vi "AO_6711_Init_Session.vi"(8 "error in (no error)":errorcluster, 9 "TRAPPING Inputs":T1={"Number of Channels"=4, "Init Values"=[2.0, 9.0, 2.0, 9.0], "Opening Values"=[0.0, 0.0, 0.0, 0.0], "Trapping Values"=[2.0, 9.0, 2.0, 9.0], "Emptying Values"=[-10.0, -10.0, -10.0, -10.0], "Adiabatic ON"=FALSE, "Adiabatic Duration"=100, "Adiabatic Waveforms"=["Adiabatic_None_2_2_2000", "Adiabatic_Ramp_9_0_2000", "Adiabatic_None_2_2_2000", "Adiabatic_RC_9_0_2000"], "Ions Refill ON"=FALSE, "Number of Ions Refills"=1} {"Number of Ions Refills" min=1 max=1000; "Trapping Values" min=-10.0 max=10.0; "Init Values" min=-10.0 max=10.0; "Emptying Values" min=-10.0 max=10.0; "Opening Values" min=-10.0 max=10.0}, 10 "AO 6711 Inputs":T2={"Physical Channels"="AO_6711/ao0:3", "Min Voltage"=-10.0, "Max Voltage"=10.0, "Trigger Source"="/AO_6711/PFI3", "Counter"="AO_6711/ctr0"} {"Max Voltage" min=-10.0 max=10.0; "Min Voltage" min=-10.0 max=10.0}, 11 "Use Software Trigger":bool) -> (0 "error out":errorcluster, 3 "Instrument handle out":refnum<k21>)   [LabVIEW 2020]
doc: "This VI inits a waveform generation session for the AO6711 board.\n1. The physical channels are selected as Analog Outputs.\n2. Init values are immediately written to the outputs.\n3. The board is inialized to wait for pulse triggers coming from an external source, i.e. the Trigger Source, and to deliver a finite number of samples.\n4. The samples have to be stored in on-board memory in a next VI."
uses:
  controls/AO_6711_Inputs.ctl
  controls/TRAPPING_Inputs.ctl
  <vilib>/DAQmx/write.llb/DAQmx Write (Analog 1D DBL NChan 1Samp).vi
  <vilib>/DAQmx/create/channels.llb/DAQmx Create Channel (AO-Voltage-Basic).vi
  <vilib>/DAQmx/miscellaneous.llb/DAQmx Fill In Error Info.vi
  <vilib>/DAQmx/configure/timing.llb/DAQmx Timing (Sample Clock).vi
  <resource>/objmgr/daqmx.rc
panel:
  # "GO_out"
  # "Gout"
  # "GI_in"
  # "Gin"
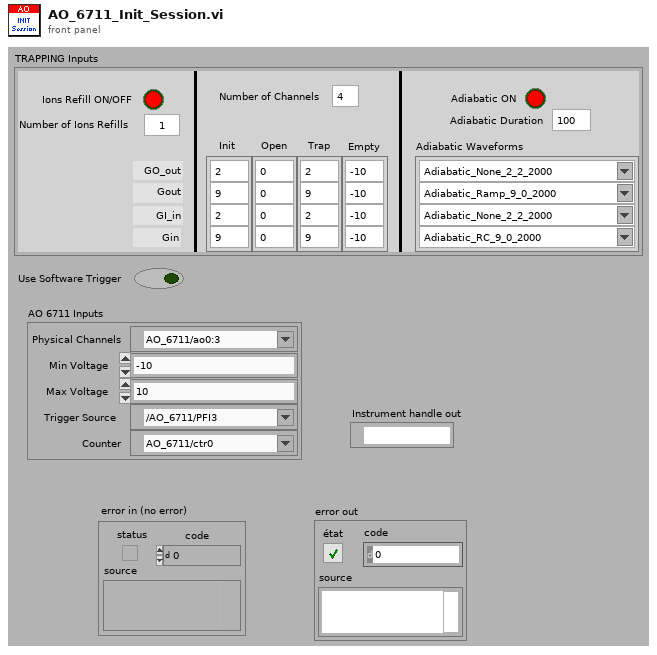
[diagram p1: front panel]
types:
  T1 = typedef "TRAPPING_Inputs.ctl" = cluster{"Number of Channels":i32, "Init Values":dbl[], "Opening Values":dbl[], "Trapping Values":dbl[], "Emptying Values":dbl[], "Adiabatic ON":bool, "Adiabatic Duration":i32, "Adiabatic Waveforms":string[], "Ions Refill ON":bool, "Number of Ions Refills":i32}
  T2 = typedef "AO_6711_Inputs.ctl" = cluster{"Physical Channels":tag, "Min Voltage":dbl, "Max Voltage":dbl, "Trigger Source":tag, "Counter":tag}
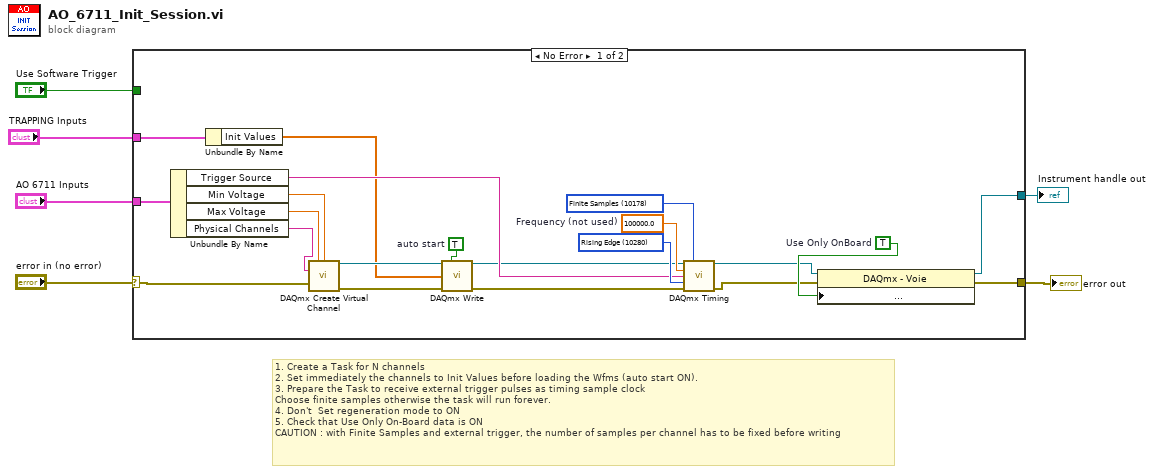
[diagram p0: block diagram]
diagram:
  # "1. Create a Task for N channels\n2. Set immediately the channels to Init Values before loading the Wfms (auto start ON).\n3. Prepare the Task to receive external trigger pulses as timing sample clock\nChoose finite samples otherwise the task will run forever.\n4. Don't  Set regeneration mode to ON\n5. Check that Use Only On-Board data is ON\nCAUTION : with Finite Samples and external trigger, the number of samples per channel has to be fixed before writing"
  n1 = case shown="No Error" "error in (no error)" {
    selector: "error in (no error)" -> [w16 w27]
    tunnel: [w13 w27] -> w6
    tunnel: "Use Software Trigger" -> [_ _]
    tunnel: [w12 _] -> w3
    tunnel: "AO 6711 Inputs" -> [w11 _]
    tunnel: "TRAPPING Inputs" -> [w10 _]
    frame No Error {
      w8 = TRUE  # auto start
      w25 = TRUE  # Use Only OnBoard
      w22 = 100000.0  # Frequency (not used)
      w21 = u16 10280 items=["Falling Edge"=10171, "Rising Edge"=10280] ("Menu déroulant")
      w26 = 10178 items=["Point par point"=12522, "Finite Samples"=10178, "Continuous Samples"=10123] ("sample mode")
      n2 = Unbundle By Name(w11) -> ("Trigger Source"=w17:tag, "Min Voltage"=w20:dbl, "Max Voltage"=w19:dbl, "Physical Channels"=w18:tag)
      n3 = Unbundle By Name(w10) -> ("Init Values"=w7:dbl[])
      n4 = call-poly <vilib>:"DAQmx Create Virtual Channel.vi"("maximum value"=w19, "minimum value"=w20, "physical channels"=w18, "error in"=w16) -> ("task out"=w15:refnum<k21>, "error out"=w14:errorcluster)  [unwired: 10 in]
      n5 = call-poly <vilib>:"DAQmx Write.vi"("task/channels in"=w15, "auto start"=w8, "data"=w7) -> ("task out"=w9:refnum<k21>)  [unwired: 10 in, 2 out]
      n6 = call-poly <vilib>:"DAQmx Timing.vi"("task/channels in"=w9, "sample mode"=w26, "rate"=w22, "source"=w17, "active edge"=w21, "error in"=w14) -> ("task out"=w24:refnum<k21>, "error out"=w23:errorcluster)  [unwired: 8 in]
      n7 = property class="DAQmx - Voie"(reference=w24, error in=w23, "Sortie analogique : Propriétés générales : Avancé : Transfert de données et mémoire : Utiliser uniquement la mémoire embarquée"=w25) -> (reference out=w12:refnum<k21>, error out=w13:errorcluster)
    }
    frame Error {
    }
  }
  "error out" <- w6
  "Instrument handle out" <- w3
